vi "main.vi"() -> ()   [LabVIEW 2021]
uses:
  <extravilib>/ChannelInstances/Stream-c(dbl,dbl)/Read With Abort.vi
  <extravilib>/ChannelInstances/Stream-c(dbl,dbl)/Write With Abort.vi
  <extravilib>/ChannelInstances/Stream-c(dbl,dbl)/EndpointRead.vi
  <extravilib>/ChannelInstances/Stream-c(dbl,dbl)/Endpoint.vi
  <vilib>/Instr/_visa.llb/VISA Configure Serial Port (Instr).vi
  <extravilib>/ChannelInstances/Event Messenger-c(str)/Instantiate.vi
  <extravilib>/ChannelInstances/Event Messenger-c(str)/))Channel.vi
  <extravilib>/ChannelInstances/Stream-c(dbl,dbl)/Instantiate.vi
  <extravilib>/ChannelInstances/Stream-c(dbl,dbl)/)Channel.vi
  <resource>/ChannelSupport/_ChannelSupport/WaitIfNeeded.vi
  <extravilib>/ChannelInstances/Stream-c(dbl,dbl).lvlib
  <extravilib>/ChannelInstances/Event Messenger-c(str).lvlib
panel:
  in  "Start":bool
  out "File Path":path
  out "Recording?":bool
  in  "Record?":bool
  out "XY Graph":cluster{"X":dbl, "Y":dbl}[](graph)
  out "Strain":dbl
  out "Time":dbl
  in  "VISA resource name":refnum<visa-resource-name>
  in  "Stop":bool
  # "Select the VISA resource name before starting the application, you can choose to record to a file at any time using the checkbox. Data acquisition begins after you press Start."
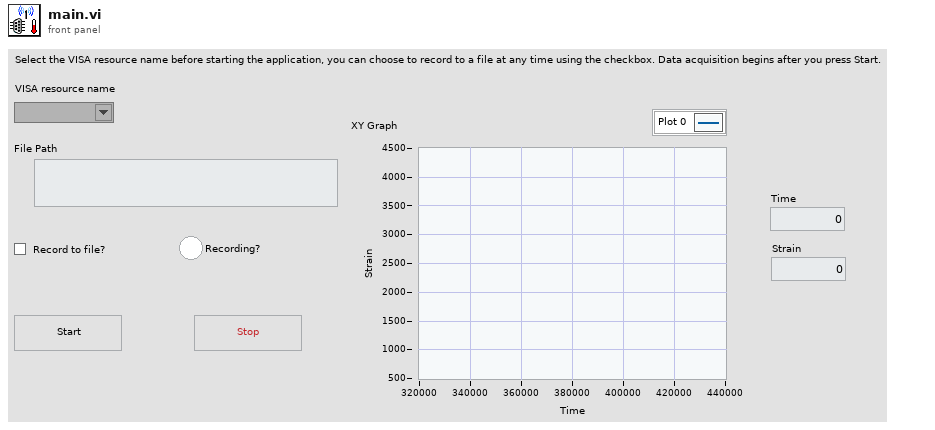
[diagram p1: front panel]
types:
  T1 = enum16{"open", "replace", "create", "open or create", "replace or create", "replace or create with confirmation"}
  T2 = typedef "Event Messenger-c(str).lvlib/))Channel.ctl" = refnum<queue>
  T3 = typedef "Stream-c(dbl,dbl).lvlib/)Channel.ctl" = refnum<queue>
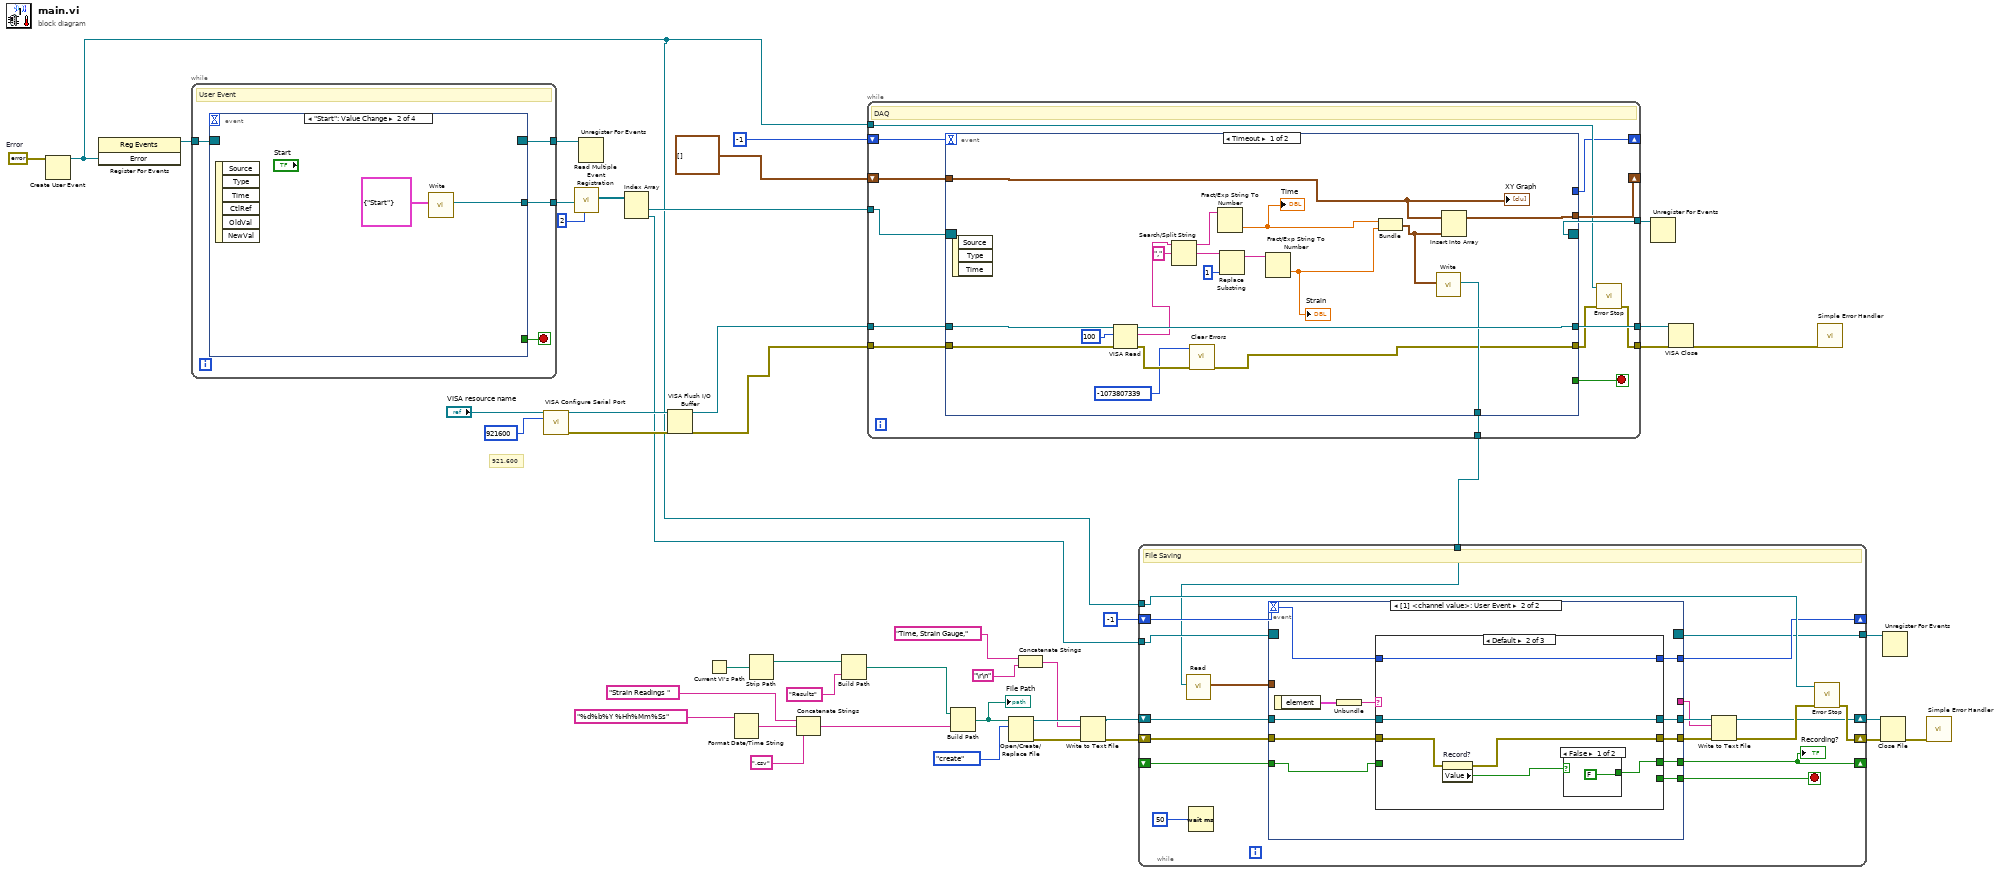
[diagram p0: block diagram]
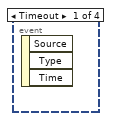
[diagram p2: hidden frame]
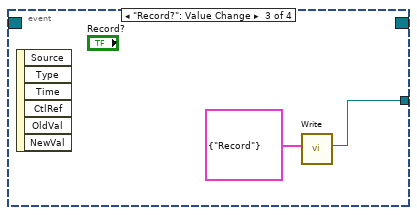
[diagram p3: hidden frame]
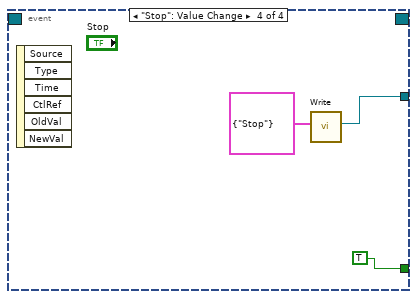
[diagram p4: hidden frame]
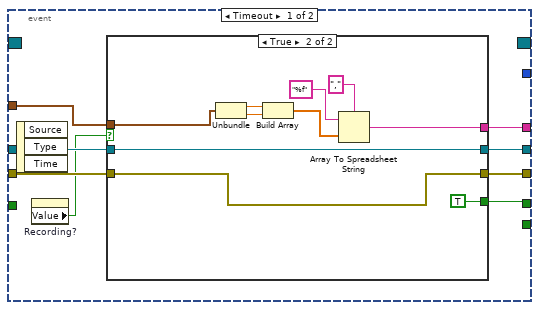
[diagram p5: hidden frame]
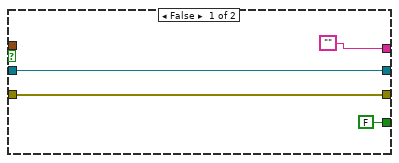
[diagram p6: hidden frame]
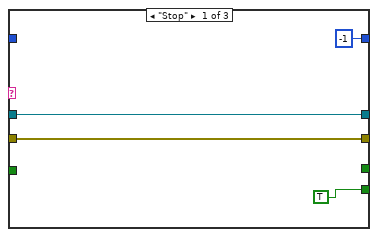
[diagram p7: hidden frame]
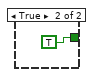
[diagram p8: hidden frame]
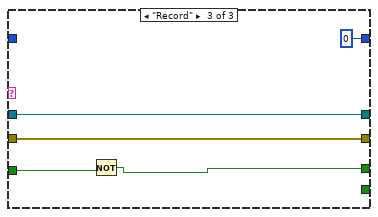
[diagram p9: hidden frame]
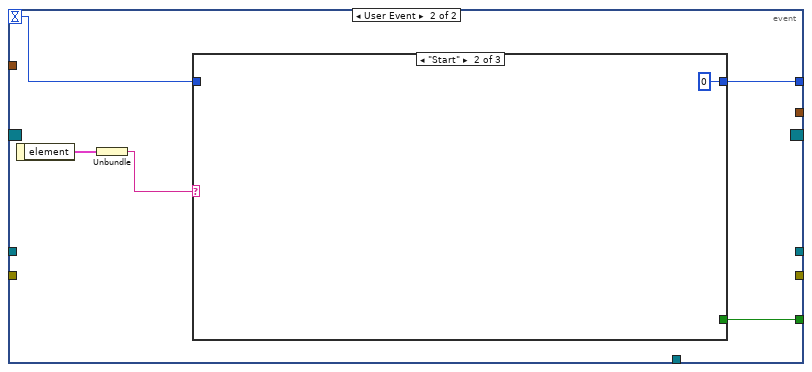
[diagram p10: hidden frame]
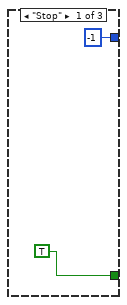
[diagram p11: hidden frame]
diagram:
  w5 = errorcluster {"status"=FALSE, "code"=0, "source"=""}  # Error
  # "921,600"
  n1 = Create User Event(user event datatype=w5) -> (user event=w4:refnum<user-event>)  [unwired: 1 in, 1 out]
  n2 = register-events(w4) -> (reference out=w15:refnum<event-registration>)  [unwired: 2 in, 1 out]
  n3 = while {
    tunnel: w15 -> [w49]
    tunnel: [w48] -> w14
    tunnel: [w47] -> w13
    stop <- w46 stop-if-true
    # "User Event"
    n4 = event shown="[1] \"Start\": Value Change" {
      selector: w49 -> [_ _ _ _]
      dyn-events: [_ _ _ _] -> w48
      timeout: _ -> [_ _ _ _]
      tunnel: [_ w50 w52 w55] -> w47
      tunnel: [_ _ _ TRUE] -> w46
      event Timeout {
        n5 = event-data() -> ()  [unwired: 1 in, 3 out]
      }
      event "Start": Value Change {
        n6 = event-data() -> ()  [unwired: 1 in, 6 out]
        n7 = call <extravilib>:"Write.vi"("element"=cluster{string} {"Start"}) -> ("channel"=w50:T2)  [unwired: 9 in, 1 out]
      }
      event "Record?": Value Change {
        n8 = event-data() -> ()  [unwired: 1 in, 6 out]
        n9 = call <extravilib>:"Write.vi"("element"=cluster{string} {"Record"}) -> ("channel"=w52:T2)  [unwired: 9 in, 1 out]
      }
      event "Stop": Value Change {
        n10 = event-data() -> ()  [unwired: 1 in, 6 out]
        n11 = call <extravilib>:"Write.vi"("element"=cluster{string} {"Stop"}) -> ("channel"=w55:T2)  [unwired: 9 in, 1 out]
      }
    }
  }
  n12 = call-poly "VISA Configure Serial Port"("VISA resource name"="VISA resource name", "baud rate (9600)"=u32 921600) -> ("VISA resource name out"=w45:refnum<visa-resource-name>, "error out"=w44:errorcluster)  [unwired: 12 in]
  n13 = call <extravilib>:"Read Multiple Event Registration.vi"("number of event structures"=u16 2, "channel"=w13) -> ("event registration refnums"=w11:refnum<event-registration>[])  [unwired: 9 in]
  n14 = Unregister For Events(event registration refnum=w14) -> ()  [unwired: 1 in, 1 out]
  n15 = Index Array(array=w11) -> (element #1=w8:refnum<event-registration>, element #2=w6:refnum<event-registration>)  [unwired: 2 in]
  n16 = VISA Flush I/O Buffer(VISA resource name=w45, error in (no error)=w44) -> (VISA resource name out=w10:refnum<visa-resource-name>, error out=w9:errorcluster)  [unwired: 1 in]
  n17 = Current VI's Path() -> (path=w33:path)
  n18 = Format Date/Time String(time format string (%c)="%d%b%Y %Hh%Mm%Ss") -> (date/time string=w37:string)  [unwired: 2 in]
  n19 = Strip Path(path=w33) -> (stripped path=w16:path)  [unwired: 1 out]
  n20 = Concatenate Strings("Strain Readings " ("string"), w37, ".csv" ("string")) -> (w35:string)
  n21 = Build Path(base path=w16, name or relative path="Results") -> (appended path=w34:path)
  n22 = while {
    tunnel: w9 -> [w70]
    tunnel: w10 -> [w69]
    tunnel: [w59] -> w42
    tunnel: [w68] -> w41
    shift-right: [w67] -> _
    shift-left: cluster{dbl, dbl}[] [] -> [w66]
    tunnel: [w65] -> w20
    tunnel: w8 -> [w64]
    tunnel: [w63] -> w7
    tunnel: w4 -> [w61]
    shift-right: [w57] -> _
    shift-left: -1 -> [w58]
    stop <- w62 stop-if-true
    # "DAQ"
    n23 = event shown="[0] Timeout" {
      selector: w64 -> [_ _]
      dyn-events: [_ _] -> w63
      timeout: w58 -> [_ w91]
      tunnel: w70 -> [w89 _]
      tunnel: w69 -> [w88 _]
      tunnel: [w87 _] -> w68
      tunnel: [w86 _] -> w67
      tunnel: w66 -> [w85 _]
      tunnel: [w84 _] -> w65
      tunnel: [w83 _] -> w60
      tunnel: [_ w92] -> w62
      tunnel: [_ w90] -> w57
      event Timeout {
        n24 = event-data() -> ()  [unwired: 1 in, 3 out]
        n25 = VISA Read(VISA resource name=w88, byte count=u32 100, error in (no error)=w89) -> (VISA resource name out=w87:refnum<visa-resource-name>, read buffer=w78:string, error out=w81:errorcluster)  [unwired: 1 out]
        n26 = Search/Split String(string=w78, search string/char (-)=",") -> (substring before match=w77:string, match + rest of string=w76:string)  [unwired: 1 in, 1 out]
        n27 = call <vilib>:"Clear Errors.vi"("error in (no error)"=w81, "specific error code to clear (0: all)"=-1073807339) -> ("error out"=w83:errorcluster)  [unwired: 4 in, 1 out]
        n28 = Fract/Exp String To Number(string=w77) -> (number=w73:dbl)  [unwired: 3 in, 1 out]
        "Time" <- w73
        n29 = Replace Substring(2:1 ("length (len. of substring)"), 5:w76) -> (1:w74:string)  [unwired: 2 in, 1 out]
        n30 = Fract/Exp String To Number(string=w74) -> (number=w72:dbl)  [unwired: 3 in, 1 out]
        "Strain" <- w72
        n31 = Bundle(w73, w72) -> (w71:cluster{dbl, dbl})  [unwired: 1 in]
        n32 = call <extravilib>:"Write.vi"("element"=w71) -> ("channel"=w84:T3)  [unwired: 8 in, 2 out]
        n33 = Insert Into Array(array=w85, new element=w71) -> (w86:cluster{dbl, dbl}[])  [unwired: 1 in]
        "XY Graph" <- w85
      }
      event User Event {
        n34 = event-data() -> ("element"=w94:cluster{string})  [unwired: 1 in]
        n35 = Unbundle(w94) -> (w93:string)
        n36 = case shown="\"Start\"" w93 {
          tunnel: [TRUE _ _] -> w92
          tunnel: w91 -> [_ _ w98]
          tunnel: [-1 0 w98] -> w90
          frame "Stop" {
          }
          frame "Start" {
          }
          frame Default {
          }
        }
      }
    }
    n37 = call "Error Stop.vi"("error in"=w60, "user event"=w61) -> ("error out"=w59:errorcluster)  [unwired: 9 in]
  }
  n38 = Build Path(base path=w34, name or relative path=w35) -> (appended path=w17:path)
  "File Path" <- w17
  n39 = Open/Create/Replace File(file path (use dialog)=w17, operation (0:open)=T1."create") -> (refnum out=w31:refnum<file>, error out=w30:errorcluster)  [unwired: 4 in, 1 out]
  n40 = Concatenate Strings("Time, Strain Gauge,", "\r\n") -> (w27:string)
  n41 = Write to Text File(file (use dialog)=w31, text=w27, error in=w30) -> (refnum out=w18:refnum<file>, error out=w25:errorcluster)  [unwired: 1 in, 1 out]
  n42 = while {
    shift-right: [w100] -> w22
    shift-left: w18 -> [w117]
    shift-right: [w113] -> w24
    shift-left: w25 -> [w116]
    tunnel: w20 -> [w106]
    tunnel: w6 -> [w115]
    tunnel: w4 -> [w114]
    shift-right: [w111] -> _
    shift-left: -1 -> [w112]
    shift-right: [w109] -> _
    shift-left: _ -> [w108]
    tunnel: [w99] -> w1
    stop <- w110 stop-if-true
    # "File Saving"
    n43 = call <extravilib>:"Read.vi"("channel"=w106) -> ("element"=w107:cluster{dbl, dbl})  [unwired: 6 in, 4 out]
    n44 = Wait (ms)(milliseconds to wait=u32 50) -> ()  [unwired: 1 out]
    n45 = event shown="[1] <channel value>: User Event" {
      selector: w115 -> [_ _]
      dyn-events: [_ _] -> w99
      timeout: w112 -> [_ w148]
      tunnel: w117 -> [w125 w141]
      tunnel: w116 -> [w124 w143]
      tunnel: [w119 w142] -> w104
      tunnel: [_ w147] -> w111
      tunnel: [_ w146] -> w110
      tunnel: [w123 w145] -> w109
      tunnel: w108 -> [_ w144]
      tunnel: w107 -> [w121 _]
      tunnel: [w120 w140] -> w102
      tunnel: [w118 _] -> w101
      event Timeout {
        n46 = event-data() -> ()  [unwired: 1 in, 3 out]
        n47 = property on="Recording?" class="Bool (strict)"() -> ("Value"=w122:bool)  [unwired: 2 in, 2 out]
        n48 = case shown="True" w122 {
          tunnel: w125 -> [w127 w132]
          tunnel: [w127 w132] -> w120
          tunnel: [w128 w131] -> w119
          tunnel: w124 -> [w128 w131]
          tunnel: [FALSE TRUE] -> w123
          tunnel: w121 -> [_ w133]
          tunnel: ["" w130] -> w118
          frame False {
          }
          frame True {
            n49 = Unbundle(w133) -> (w139:dbl, w138:dbl)
            n50 = Build Array(w139, w138) -> (w135:dbl[])
            n51 = Array To Spreadsheet String(delimiter (Tab)=",", array=w135, 3:"%f" ("format string")) -> (spreadsheet string=w130:string)
          }
        }
      }
      event User Event {
        n52 = event-data() -> ("element"=w150:cluster{string})  [unwired: 1 in]
        n53 = Unbundle(w150) -> (w149:string)
        n54 = case shown="Default" w149 {
          tunnel: w148 -> [_ w160 _]
          tunnel: [-1 w160 0] -> w147
          tunnel: [TRUE _ _] -> w146
          tunnel: [_ w155 w165] -> w145
          tunnel: w144 -> [_ _ w166]
          tunnel: w143 -> [w152 w158 w164]
          tunnel: [w152 w157 w164] -> w142
          tunnel: w141 -> [w151 w159 w163]
          tunnel: [w151 w159 w163] -> w140
          frame "Stop" {
          }
          frame Default {
            n55 = property on="Record?" class="Bool (strict)"(error in=w158) -> (error out=w157:errorcluster, "Value"=w156:bool)  [unwired: 1 in, 1 out]
            n56 = case shown="False" w156 {
              tunnel: [FALSE TRUE] -> w155
              frame False {
              }
              frame True {
              }
            }
          }
          frame "Record" {
            n57 = Not(x=w166) -> (.not. x?=w165:bool)
          }
        }
      }
    }
    "Recording?" <- w109
    n58 = Write to Text File(file (use dialog)=w102, text=w101, error in=w104) -> (refnum out=w100:refnum<file>, error out=w103:errorcluster)  [unwired: 1 in, 1 out]
    n59 = call "Error Stop.vi"("error in"=w103, "user event"=w114) -> ("error out"=w113:errorcluster)  [unwired: 9 in]
  }
  n60 = Unregister For Events(event registration refnum=w7) -> ()  [unwired: 1 in, 1 out]
  n61 = VISA Close(VISA resource name=w41, error in (no error)=w42) -> (error out=w40:errorcluster)
  n62 = call <vilib>:"Simple Error Handler.vi"("error in (no error)"=w40) -> ()  [unwired: 4 in, 5 out]
  n63 = Close File(refnum=w22, error in=w24) -> (error out=w23:errorcluster)  [unwired: 1 out]
  n64 = Unregister For Events(event registration refnum=w1) -> ()  [unwired: 1 in, 1 out]
  n65 = call <vilib>:"Simple Error Handler.vi"("error in (no error)"=w23) -> ()  [unwired: 4 in, 5 out]
